vi "Set Inline Buffer.vi"(8 "error in (no error)":errorcluster, 10 "base Inline Buffer":refnum<class "Buffer.lvclass">, 11 "Data Server Thread in":refnum<class "Data Server Thread.lvclass">) -> (0 "error out":errorcluster, 3 "Data Server Thread out":refnum<class "Data Server Thread.lvclass">)   [LabVIEW 2019, in "DSF Core.lvlib" / "Data Server Thread.lvclass"]
uses:
  Data Server Thread.lvclass
  Buffer/Buffer.lvclass
  Data Server Thread.lvclass/Data Server Thread.ctl
  Transfer/Transfer.lvclass
  Buffers/Buffers.lvclass
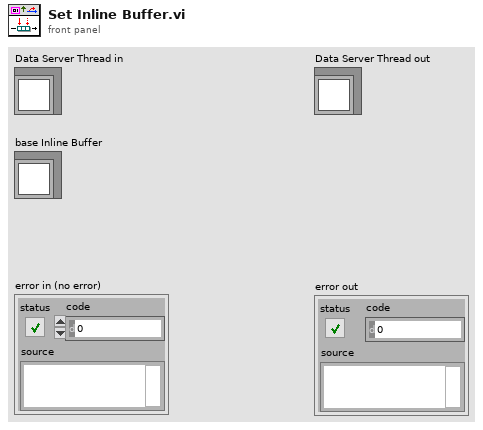
[diagram p1: front panel]
types:
  T1 = typedef "DSF Core.lvlib/Data Server Thread.lvclass/Plugin.ctl" = cluster{"Plugin Status":refnum<class "Status Pointer.lvclass">, "Groups":T2[]}
  T2 = typedef "DSF Core.lvlib/Data Server Thread.lvclass/Group.ctl" = cluster{"Group Buffers":refnum<class "Buffers.lvclass">, "Group Status":refnum<class "Status Pointer.lvclass">, "Transfers":refnum<class "Transfer.lvclass">[]}
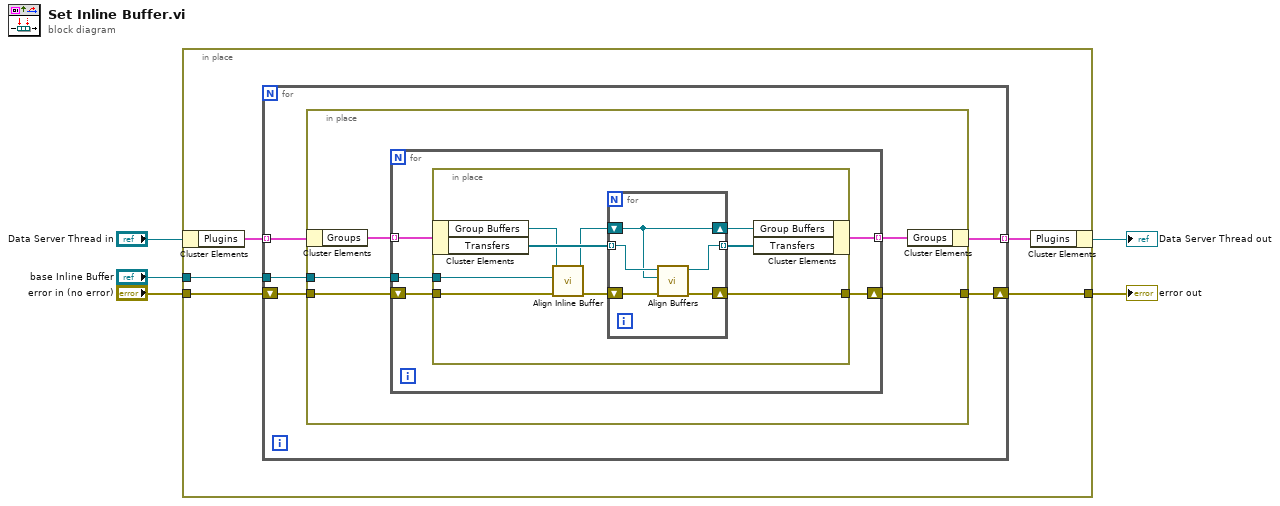
[diagram p0: block diagram]
diagram:
  n1 = in-place {
    in-place-border: "base Inline Buffer" -> [w9]
    in-place-border: "error in (no error)" -> [w8]
    in-place-border: [w7] -> w1
    n2 = in-place-cluster #1("Data Server Thread in") -> ("Plugins"=w10:T1[])
    n3 = for {
      tunnel: w10 -> [w12] mode=indexing
      tunnel: w9 -> [w15]
      shift-right: [w13] -> w7
      shift-left: w8 -> [w14]
      tunnel: [w11] -> w6 mode=indexing
      n4 = in-place {
        in-place-border: w15 -> [w16]
        in-place-border: w14 -> [w17]
        in-place-border: [w20] -> w13
        n5 = in-place-cluster #2(w12) -> ("Groups"=w19:T2[])
        n6 = for {
          tunnel: w19 -> [w23] mode=indexing
          tunnel: w16 -> [w22]
          shift-right: [w24] -> w20
          shift-left: w17 -> [w25]
          tunnel: [w21] -> w18 mode=indexing
          n7 = in-place {
            in-place-border: w25 -> [w27]
            in-place-border: [w34] -> w24
            in-place-border: w22 -> [w28]
            n8 = in-place-cluster #3(w23) -> ("Group Buffers"=w30:refnum<class "Buffers.lvclass">, "Transfers"=w33:refnum<class "Transfer.lvclass">[])
            n9 = call "Align Inline Buffer.vi"("error in (no error)"=w27, "base Inline Buffer"=w28, "Buffers in"=w30) -> ("error out"=w26:errorcluster, "Buffers out"=w29:refnum<class "Buffers.lvclass">)  [unwired: 7 in]
            n10 = for {
              tunnel: w33 -> [w39] mode=indexing
              tunnel: [w36] -> w31 mode=indexing
              shift-right: [w37] -> w34
              shift-left: w26 -> [w38]
              shift-right: [w35] -> w32
              shift-left: w29 -> [w35]
              n11 = call "Align Buffers.vi"("error in (no error)"=w38, "Transfer Group Buffers"=w35, "Transfer in"=w39) -> ("error out"=w37:errorcluster, "Transfer out"=w36:refnum<class "Transfer.lvclass">)  [unwired: 7 in]
            }
            n12 = in-place-cluster #3("Group Buffers"=w32, "Transfers"=w31) -> (w21:T2)
          }
        }
        n13 = in-place-cluster #2("Groups"=w18) -> (w11:T1)
      }
    }
    n14 = in-place-cluster #1("Plugins"=w6) -> (→"Data Server Thread out":refnum<class "Data Server Thread.lvclass">)
  }
  "error out" <- w1
